vi "Back_End_Chiller_PID.vi"(1 "Present Value":dbl=15.0 format="%.2f", 2 "Previous Control Sum":dbl format="%.2f", 3 "Setpoint":dbl=15.0 format="%.2f") -> (0 "Dem Output":dbl format="%.2f")   [LabVIEW 2016]
uses:
  <vilib>/Analysis/NI_AALPro.lvlib
panel:
  out "Derivative":dbl(graph)
  out "Integral":dbl(graph)
  out "Proportional":dbl(graph)
  out "Error":dbl(graph)
  in  "O/P deadband":dbl=1.0 format="%.2f"
  in  "Kp Deadband":dbl format="%.2f"
  in  "Derivative History":i32=20
  out "deadbanded error":dbl format="%.2f"
  in  "P":bool=TRUE
  in  "D":bool=TRUE
  in  "I":bool=TRUE
  in  "Manual Demand":dbl min=0.0 max=100.0 format="%.2f"
  in  "Manual Override":bool
  out "Control Sum":dbl format="%.2f"
  out "error differential":dbl format="%.5f"
  out "error integral":dbl format="%.2f"
  in  "Kd":dbl=25.0 format="%.2f"
  in  "Ki":dbl=0.1 format="%.3f"
  in  "Kp":dbl=10.0 format="%.2f"
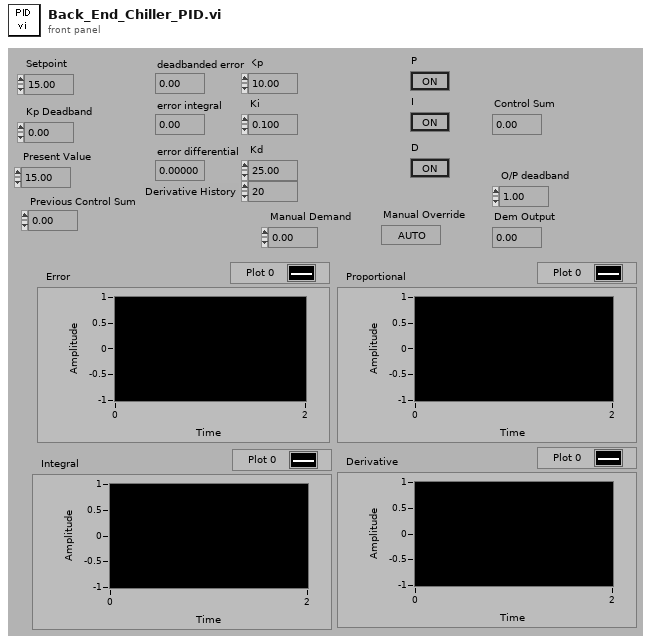
[diagram p1: front panel]
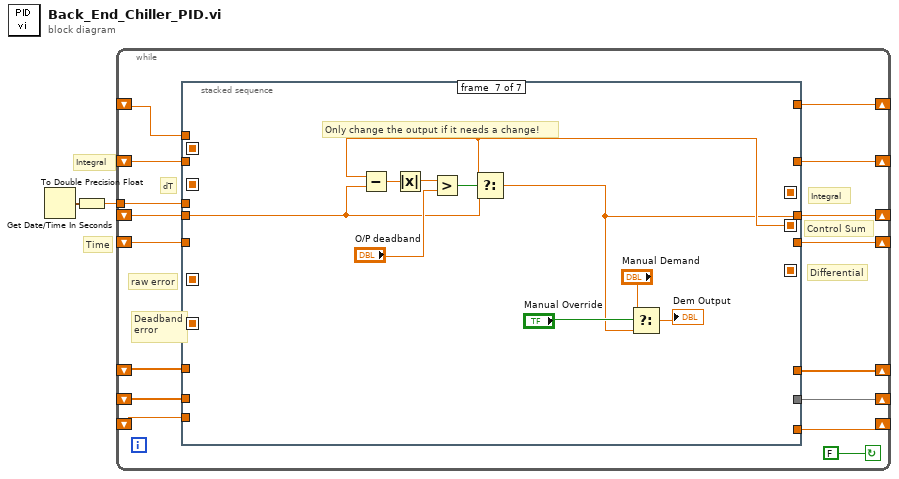
[diagram p0: block diagram]
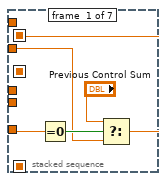
[diagram p2: hidden frame]
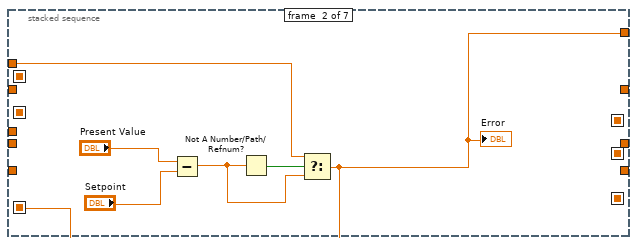
[diagram p3: hidden frame]
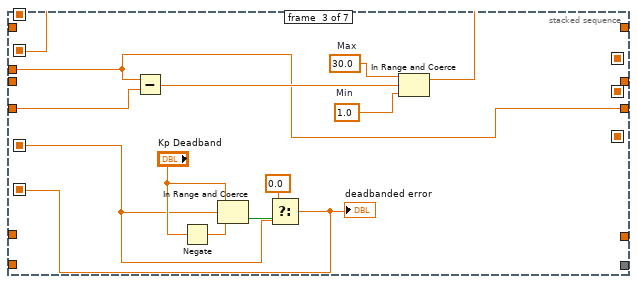
[diagram p4: hidden frame]
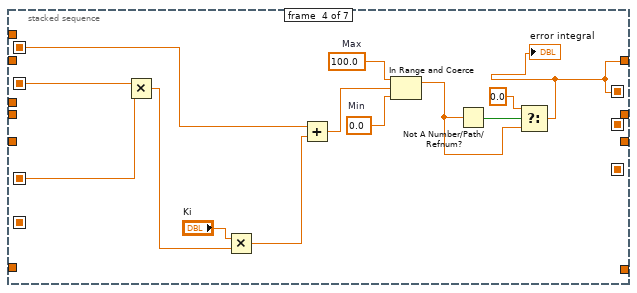
[diagram p5: hidden frame]
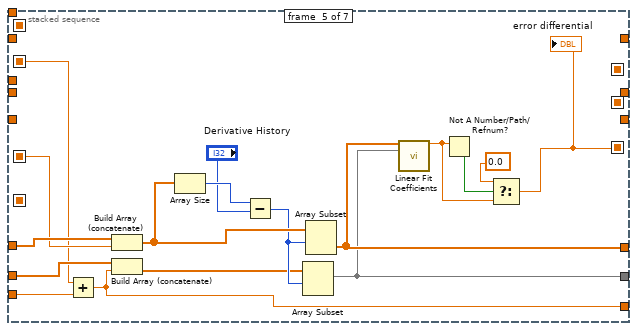
[diagram p6: hidden frame]
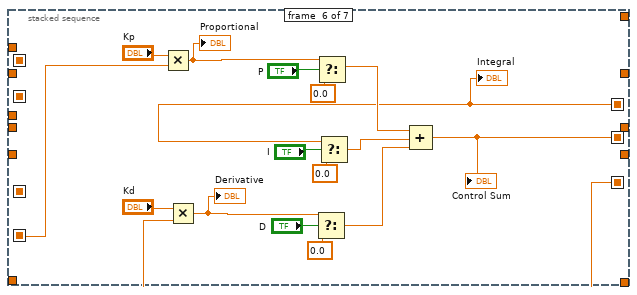
[diagram p7: hidden frame]
diagram:
  # "Integral"
  # "Time"
  n1 = Get Date/Time In Seconds() -> (seconds since 1Jan1904=w1:timestamp)
  n2 = To Double Precision Float(number=w1) -> (double precision float=w2:dbl)
  n3 = while {
    shift-left: _ -> [w5]
    shift-right: [w4] -> _
    shift-left: _ -> [w7]
    shift-right: [w6] -> _
    shift-left: _ -> [w9]
    shift-right: [w8] -> _
    tunnel: w2 -> [w14]
    shift-left: _ -> [w11]
    shift-right: [w10] -> _
    shift-left: _ -> [w13]
    shift-right: [w12] -> _
    shift-left: _ -> [w15]
    shift-right: [w16] -> _
    shift-left: _ -> [w18]
    shift-right: [w17] -> _
    stop <- FALSE continue-if-true
    # "Control Sum"
    # "raw error"
    # "Differential"
    # "Integral"
    # "Deadband\nerror"
    # "dT"
    n4 = stacked-sequence {
      seq-local: [_ _ w30 _ _ _ _] -> [_ _ _ w54 w57 _ _]
      seq-local: [_ _ w39 _ _ _ _] -> [_ _ _ _ _ w76 _]
      seq-local: [_ _ _ _ w62 _ _] -> [_ _ _ _ _ w75 _]
      seq-local: [_ _ _ w47 _ _ _] -> [_ _ _ _ _ w74 _]
      seq-local: [_ w24 _ _ _ _ _] -> [_ _ w31 w51 w63 _ _]
      seq-local: [_ _ _ _ _ w79 _] -> [_ _ _ _ _ _ w92]
      seq-local: [w19 _ _ _ _ _ _] -> [_ _ _ w44 _ _ _]
      tunnel: w18 -> [w23 _ w36 _ _ _ _]
      tunnel: [_ _ w34 _ _ _ _] -> w17
      tunnel: [_ _ _ w47 _ _ _] -> w16
      tunnel: w15 -> [w20 _ _ _ _ _ _]
      tunnel: w14 -> [_ _ w34 _ _ _ _]
      tunnel: w13 -> [_ _ _ _ w71 _ _]
      tunnel: [_ _ _ _ w64 _ _] -> w12
      tunnel: w11 -> [_ _ _ _ w70 _ _]
      tunnel: [_ _ _ _ w61 _ _] -> w10
      tunnel: w9 -> [_ _ _ _ _ _ w90]
      tunnel: [_ _ _ _ _ _ w89] -> w8
      tunnel: w7 -> [_ _ _ _ w56 _ _]
      tunnel: [_ _ _ _ w55 _ _] -> w6
      tunnel: w5 -> [_ w26 _ _ _ _ _]
      tunnel: [_ w24 _ _ _ _ _] -> w4
      frame #0 {
        n5 = Equal To 0?(x=w23) -> (x = 0?=w22:bool)
        n6 = Select(t="Previous Control Sum", s=w22, f=w20) -> (s? t:f=w19:dbl)
      }
      frame #1 {
        n7 = Subtract(x="Present Value", y="Setpoint") -> (x-y=w25:dbl)
        n8 = Not A Number/Path/Refnum?(number/path/refnum=w25) -> (NaN/Path/Refnum?=w27:bool)
        n9 = Select(t=w26, s=w27, f=w25) -> (s? t:f=w24:dbl)
        "Error" <- w24
      }
      frame #2 {
        w37 = 1.0  # Min
        w38 = 30.0  # Max
        n10 = Subtract(x=w34, y=w36) -> (x-y=w35:dbl)
        n11 = Negate(x="Kp Deadband") -> (-x=w33:dbl)
        n12 = In Range and Coerce(upper limit="Kp Deadband", x=w31, lower limit=w33) -> (In Range?=w40:bool)  [unwired: 1 out]
        n13 = Select(t=0.0, s=w40, f=w31) -> (s? t:f=w39:dbl)
        "deadbanded error" <- w39
        n14 = In Range and Coerce(upper limit=w38, x=w35, lower limit=w37) -> (coerced(x)=w30:dbl)  [unwired: 1 out]
      }
      frame #3 {
        w53 = 0.0  # Min
        w42 = 100.0  # Max
        n15 = Multiply(x=w54, y=w51) -> (x*y=w45:dbl)
        n16 = Multiply(x="Ki", y=w45) -> (x*y=w43:dbl)
        n17 = Add(x=w44, y=w43) -> (x+y=w52:dbl)
        n18 = In Range and Coerce(upper limit=w42, x=w52, lower limit=w53) -> (coerced(x)=w48:dbl)  [unwired: 1 out]
        n19 = Not A Number/Path/Refnum?(number/path/refnum=w48) -> (NaN/Path/Refnum?=w49:bool)
        n20 = Select(t=0.0, s=w49, f=w48) -> (s? t:f=w47:dbl)
        "error integral" <- w47
      }
      frame #4 {
        n21 = Add(x=w57, y=w56) -> (x+y=w55:dbl)
        n22 = Build Array (concatenate)(w71, w63) -> (w67:dbl[])
        n23 = Build Array (concatenate)(w70, w55) -> (w65:dbl[])
        n24 = Array Size(array=w67) -> (size(s)=w69:i32)
        n25 = Subtract(x=w69, y="Derivative History") -> (x-y=w66:i32)
        n26 = Array Subset(array=w65, index=w66) -> (w61:dbl[])  [unwired: 1 in]
        n27 = Array Subset(array=w67, index=w66) -> (w64:dbl[])  [unwired: 1 in]
        n28 = call <vilib>:"Linear Fit Coefficients.vi"("Y"=w64, "X"=w61) -> ("slope"=w58:dbl)  [unwired: 3 in, 10 out]
        n29 = Not A Number/Path/Refnum?(number/path/refnum=w58) -> (NaN/Path/Refnum?=w60:bool)
        n30 = Select(t=0.0 ("f"), s=w60, f=w58) -> (s? t:f=w62:dbl)
        "error differential" <- w62
      }
      frame #5 {
        n31 = Multiply(x="Kp", y=w76) -> (x*y=w72:dbl)
        "Proportional" <- w72
        n32 = Multiply(x="Kd", y=w75) -> (x*y=w73:dbl)
        "Derivative" <- w73
        n33 = Select(t=w73, s="D", f=0.0) -> (s? t:f=w81:dbl)
        n34 = Select(t=w72, s="P", f=0.0) -> (s? t:f=w87:dbl)
        n35 = Select(t=w74, s="I", f=0.0) -> (s? t:f=w80:dbl)
        n36 = Compound Arithmetic op=ADD(w87, w80, w81) -> (w79:dbl)
        "Control Sum" <- w79
        "Integral" <- w74
      }
      frame #6 {
        # "Only change the output if it needs a change!"
        n37 = Subtract(x=w92, y=w90) -> (x-y=w95:dbl)
        n38 = Absolute Value(x=w95) -> (abs(x)=w94:dbl)
        n39 = Greater?(x=w94, y="O/P deadband") -> (0:w93:bool)
        n40 = Select(t=w92, s=w93, f=w90) -> (s? t:f=w89:dbl)
        n41 = Select(t="Manual Demand", s="Manual Override", f=w89) -> (s? t:f=→"Dem Output":dbl)
      }
    }
  }
